vi "queue_gui.vi"(6 "QueueActions":T3, 8 "error in (no error)":errorcluster, 10 "QueueDataIn":T1) -> (0 "error out":errorcluster, 3 "queue out":refnum<queue>)   [LabVIEW 2020]
uses:
  #typedefs/#typedef_enum_QueueActions.ctl
  #typedefs/#typedef_cluster_GUI_QueueData.ctl
  #typedefs/#typedef_enum_GUI_States.ctl
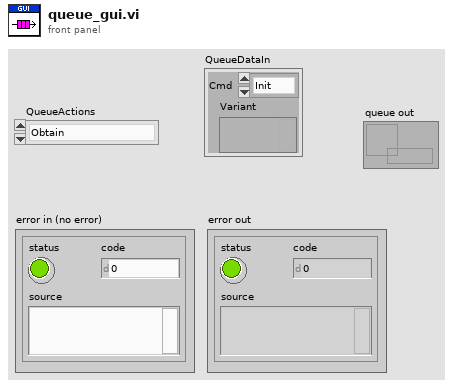
[diagram p1: front panel]
types:
  T1 = typedef "#typedef_cluster_GUI_QueueData.ctl" = cluster{"Cmd":T2, "Variant":variant}
  T2 = typedef "#typedef_enum_GUI_States.ctl" = enum16{"Init", "AddImages", "PreviousImage", "NextImage", "AnalyzeImage", "SaveImage", "GenFakeError", "ErrorHandling", "ExitRequest", "Exit"}
  T3 = typedef "#typedef_enum_QueueActions.ctl" = enum16{"Obtain", "GetRef", "Enqueue", "Release"}
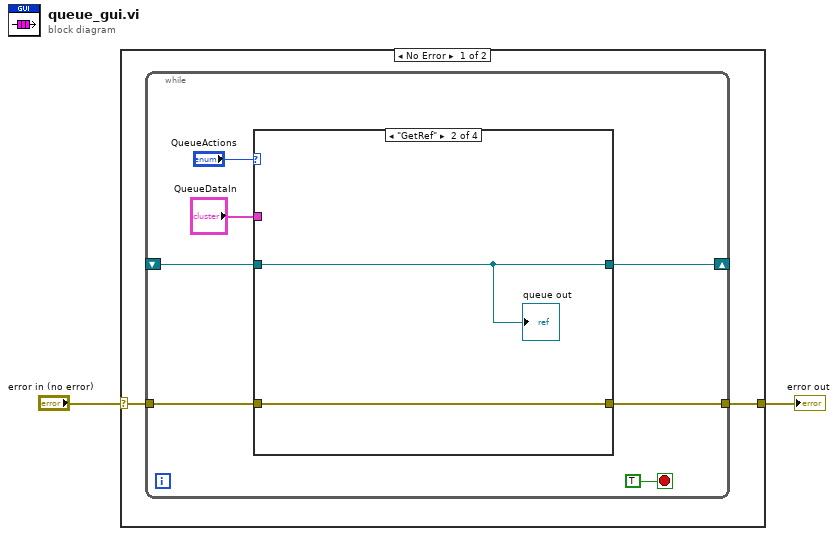
[diagram p0: block diagram]
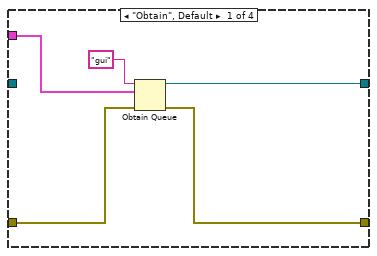
[diagram p2: hidden frame]
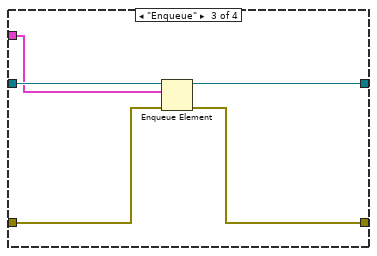
[diagram p3: hidden frame]
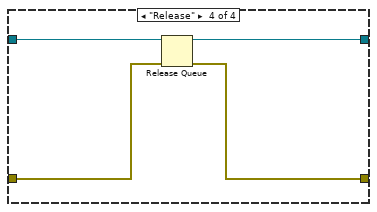
[diagram p4: hidden frame]
diagram:
  n1 = case shown="No Error" "error in (no error)" {
    selector: "error in (no error)" -> [w4 w27]
    tunnel: [w3 w27] -> w1
    frame No Error {
      n2 = while {
        shift-right: [w7] -> _
        shift-left: _ -> [w6]
        tunnel: w4 -> [w9]
        tunnel: [w8] -> w3
        stop <- TRUE stop-if-true
        n3 = case shown="\"GetRef\"" "QueueActions" {
          tunnel: w9 -> [w15 w17 w23 w26]
          tunnel: [w14 w17 w22 w25] -> w8
          tunnel: [w13 w18 w19 w24] -> w7
          tunnel: w6 -> [_ w18 w21 w24]
          tunnel: "QueueDataIn" -> [w12 _ w20 _]
          frame "Obtain", Default {
            n4 = Obtain Queue(name (unnamed)="gui", element data type=w12, error in (no error)=w15) -> (queue out=w13:refnum<queue>, error out=w14:errorcluster)  [unwired: 2 in, 1 out]
          }
          frame "GetRef" {
            "queue out" <- w18
          }
          frame "Enqueue" {
            n5 = Enqueue Element(queue=w21, element=w20, error in (no error)=w23) -> (queue out=w19:refnum<queue>, error out=w22:errorcluster)  [unwired: 1 in, 1 out]
          }
          frame "Release" {
            n6 = Release Queue(queue=w24, error in (no error)=w26) -> (error out=w25:errorcluster)  [unwired: 1 in, 2 out]
          }
        }
      }
    }
    frame Error {
    }
  }
  "error out" <- w1
